vi "IntoExcel.vi"(0 "Array":i32[][](array[numeric]), 1 "Y Vector":dbl[](array[numeric]), 2 "X Vector":dbl[](array[numeric])) -> ()   [LabVIEW 2014]
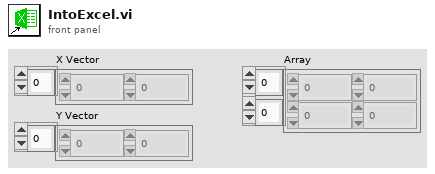
[diagram p1: front panel]
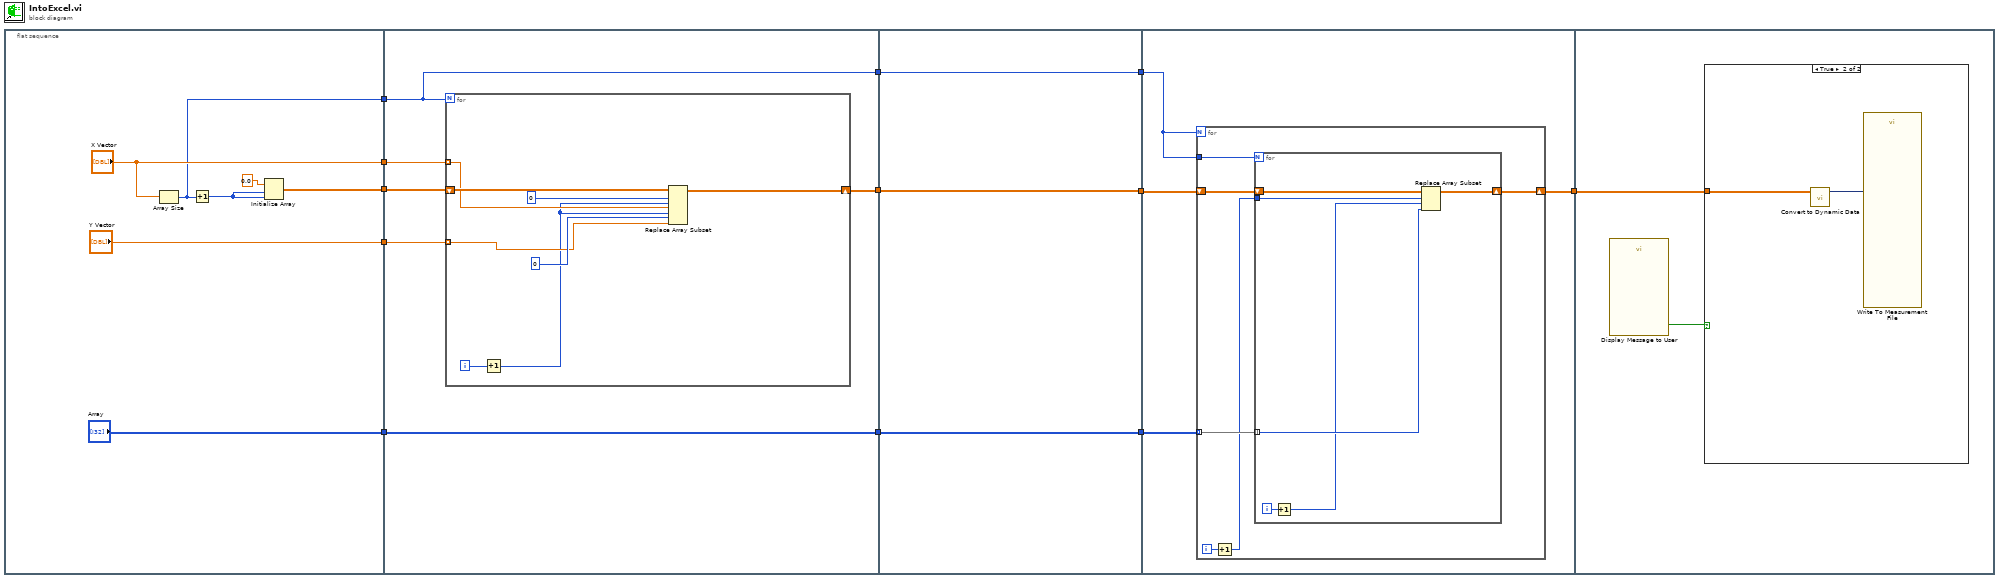
[diagram p0: block diagram]
diagram:
  n1 = flat-sequence {
    tunnel: ["Array"] -> w12
    tunnel: ["Y Vector"] -> w11
    tunnel: ["X Vector"] -> w10
    tunnel: [w16] -> w9
    tunnel: [w13] -> w8
    tunnel: w12 -> [w20]
    tunnel: w11 -> [w23]
    tunnel: w10 -> [w24]
    tunnel: w9 -> [w25]
    tunnel: w8 -> [w21]
    tunnel: [w22] -> w7
    tunnel: [w21] -> w5
    tunnel: [w20] -> w3
    tunnel: w7 -> [w34]
    tunnel: [w34] -> w6
    tunnel: w5 -> [w36]
    tunnel: [w36] -> w4
    tunnel: w3 -> [w35]
    tunnel: [w35] -> w2
    tunnel: w6 -> [w38]
    tunnel: w4 -> [w39]
    tunnel: w2 -> [w40]
    tunnel: [w37] -> w1
    tunnel: w1 -> [w53]
    frame #0 {
      n2 = Array Size(array="X Vector") -> (size(s)=w13:i32)
      n3 = Increment(x=w13) -> (x+1=w14:i32)
      n4 = Initialize Array(0.0, w14, w14) -> (w16:dbl[][])
    }
    frame #1 {
      n5 = for {
        N: w21 -> [_]
        tunnel: w24 -> [w29] mode=indexing
        tunnel: w23 -> [w30] mode=indexing
        shift-right: [w26] -> w22
        shift-left: w25 -> [w33]
        i -> [w28]
        n6 = Increment(x=w28) -> (x+1=w27:i32)
        n7 = Replace Array Subset(array=w33, new element #1=w29, index (row) #1=0 ("index (row)"), index (col) #1=w27, new element #2=w30, index (row) #2=w27, index (col) #2=0 ("disabled index (col)")) -> (w26:dbl[][])
      }
    }
    frame #2 {
    }
    frame #3 {
      n8 = for {
        N: w39 -> [_]
        tunnel: w40 -> [w44] mode=indexing
        tunnel: w39 -> [w46]
        shift-right: [w43] -> w37
        shift-left: w38 -> [w45]
        i -> [w42]
        n9 = Increment(x=w42) -> (x+1=w41:i32)
        n10 = for {
          N: w46 -> [_]
          tunnel: w44 -> [w49] mode=indexing
          tunnel: w41 -> [w51]
          shift-right: [w50] -> w43
          shift-left: w45 -> [w52]
          i -> [w48]
          n11 = Increment(x=w48) -> (x+1=w47:i32)
          n12 = Replace Array Subset(array=w52, new element=w49, index (row)=w51, index (col)=w47) -> (w50:dbl[][])
        }
      }
    }
    frame #4 {
      n13 = call "Display Message to User"() -> ("OK"=w54:bool)  [unwired: 10 in, 1 out]
      n14 = case shown="True" w54 {
        tunnel: w53 -> [_ w56]
        frame False {
        }
        frame True {
          n15 = call "Convert to Dynamic Data"("2D Array"=w56) -> ("Dynamic Data Type"=w55:dynamicdata)  [unwired: 3 in]
          n16 = call "Write To Measurement File"("Signals"=w55) -> ()  [unwired: 16 in, 3 out]
        }
      }
    }
  }
